vi "Accelerometer plot.vi"(0 "Refnum in":refnum<k20>, 1 "Ring Refnum":refnum<vi>, 4 "Host Loop update rate (ms)":u32=100, 5 "stop":bool, 7 "error in (no error)":errorcluster) -> (8 "size(s)":i32, 9 "element":dbl, 11 "Spool x acceleration":dbl, 12 "acceleration v time":waveform(dbl)[](graph), 13 "rotational speed (rpm)":dbl, 14 "Open Loop":bool[](array[boolean]), 15 "Elements Remaining":u32, 16 "Short Circuit":bool[](array[boolean]), 17 "Waveform Graph":waveform(dbl)[](graph), 18 "Spool y acceleration":dbl, 19 "Array":dbl[][](array[numeric]), 20 "Refnum out":refnum<k20>, 21 "error out":errorcluster, 23 "magnitudes":cluster{"f0":dbl, "df":dbl, "magnitude":dbl[]}[](graph), 24 "Data FIFO Full":bool, 25 "result":bool, 27 "error out":errorcluster)   [LabVIEW 2017]
uses:
  <vilib>/Analysis/4window.llb/windowTd.ctl
  <vilib>/Utility/error.llb/Error Cluster From Error Code.vi
  <vilib>/rvi/errors/niLvFpgaAdjustHostInterfaceError.vi
  <vilib>/measure/maspectr.llb/FFT Spectrum (Mag-Phase) for N Chan.vi
  <vilib>/measure/mamon.llb/Waveform Peak Detection for 1 Chan.vi
  <vilib>/rvi/interface/nirviMethod/nirviMethod.xnode
  <vilib>/rvi/interface/nirviReadWriteControl/nirviReadWriteControl.xnode
  NiFpgaLv.dll
  <vilib>/rvi/interface/Simulation/niFpgaSimulationCallBeginRW.vi
  <vilib>/FPGAPlugInAG/Dynamic/niLvFpga_ReadFifo_Dynamic.vi
  <vilib>/rvi/errors/niLvFpgaMergeErrorWithErrorCode.vi
  <vilib>/measure/NI_MAPro.lvlib
  <vilib>/Analysis/NI_AALPro.lvlib
  <vilib>/Analysis/NI_AAL_SigProc.lvlib
panel:
  out "appended array 2":waveform(dbl)[](array[waveform])
  out "appended array":waveform(dbl)[](array[waveform])
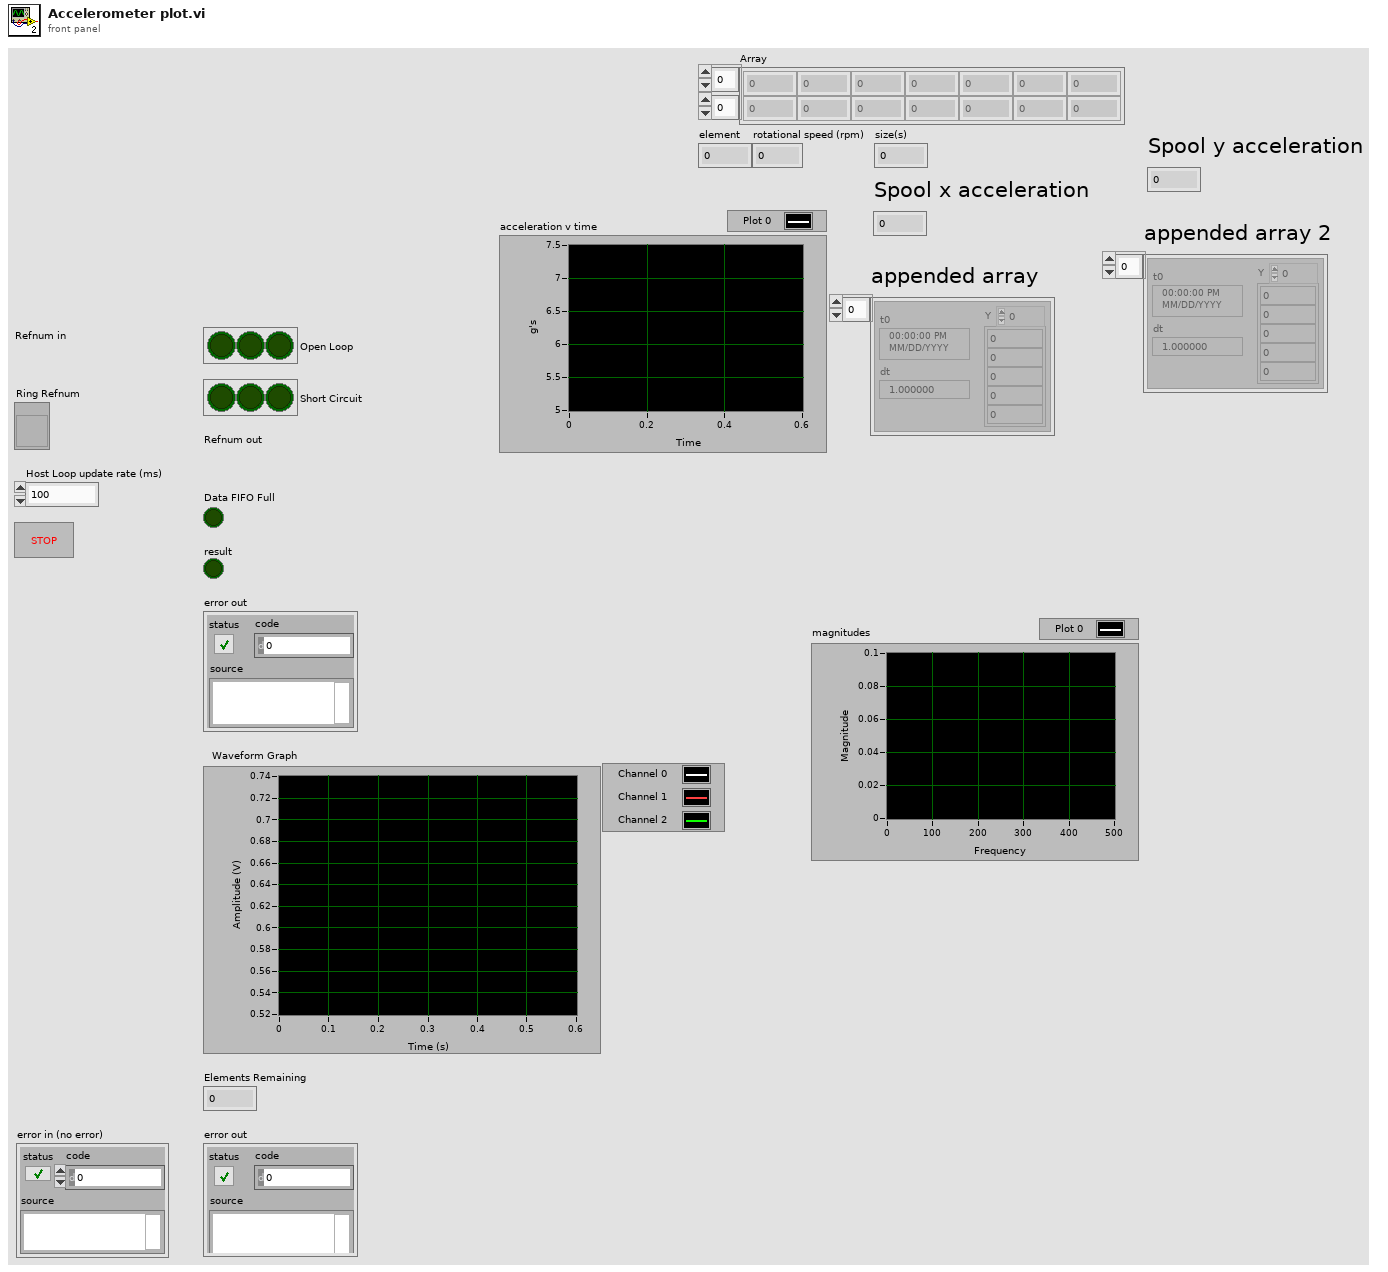
[diagram p1: front panel]
types:
  T1 = typedef "NI_AALPro.lvlib/windowTd.ctl" = u32
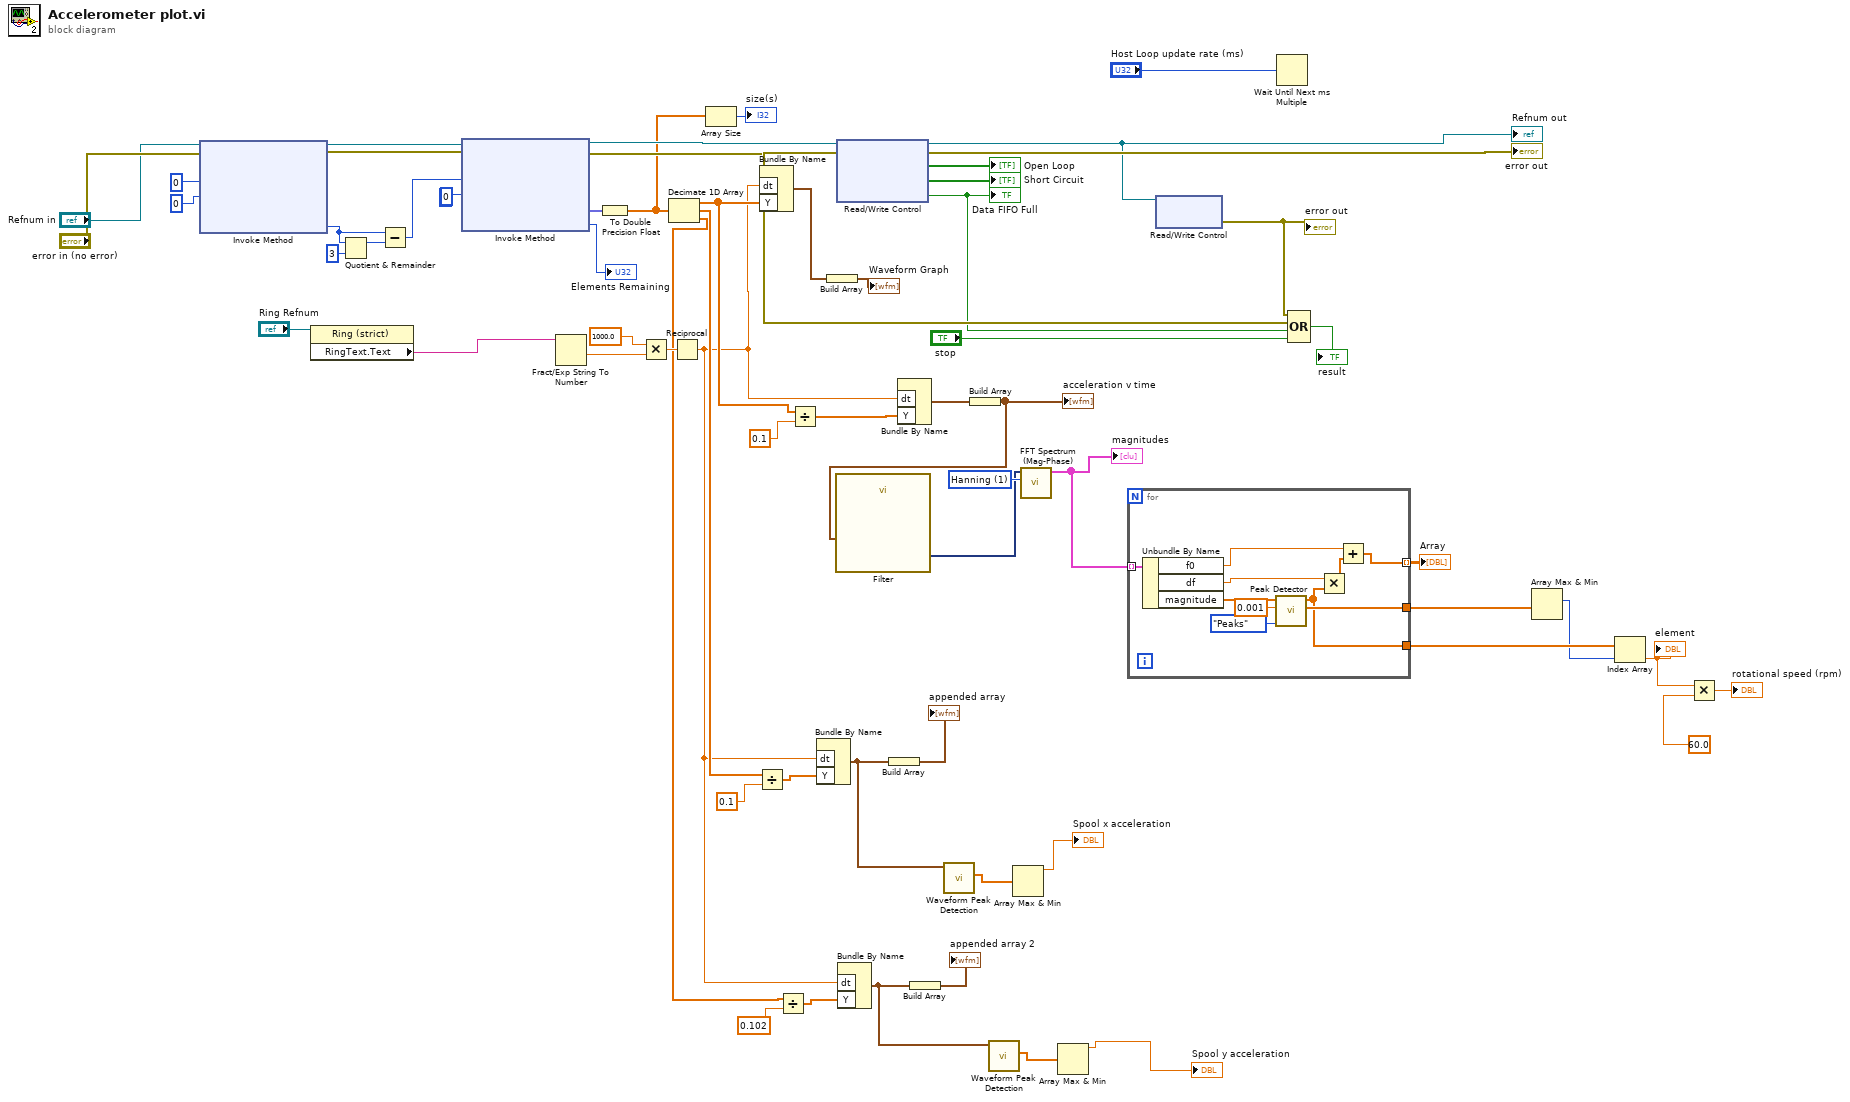
[diagram p0: block diagram]
diagram:
  w29 = T1 1 items=["Rectangle"=0, "Hanning"=1, "Hamming"=2, "Blackman-Harris"=3, "Exact Blackman"=4, "Blackman"=5, "Flat Top"=6, "4 Term B-Harris "=7, "7 Term B-Harris"=8, "Low Sidelobe"=9, "Blackman Nuttall"=11, "Triangle"=30, "Bartlett-Hanning"=31, "Bohman"=32, "Parzen"=33, "Welch"=34, "Kaiser"=60, "Dolph-Chebyshev"=61, "Gaussian"=62] ("window")
  (unwired) 0 ("Timeout")
  n1 = xnode "Invoke Method"("FPGA VI Reference In"="Refnum in", "error in"="error in (no error)", "Number of Elements"=u32 0, "Timeout (ms)"=0) -> ("FPGA VI Reference Out"=w49:refnum<k20>, "error out"=w50:errorcluster, "Elements Remaining"=w58:u32)  [unwired: 1 out]
  n2 = property on="Property Node" class="Ring (strict)"(reference="Ring Refnum") -> ("RingText.Text"=w63:string)  [unwired: 1 in, 2 out]
  n3 = Quotient & Remainder(x=w58, y=u32 3) -> (x-y*floor(x/y)=w47:u32)  [unwired: 1 out]
  n4 = Subtract(x=w58, y=w47) -> (x-y=w59:u32)
  n5 = xnode "Invoke Method"("FPGA VI Reference In"=w49, "error in"=w50, "Number of Elements"=w59, "Timeout (ms)"=0) -> ("FPGA VI Reference Out"=w40:refnum<k20>, "error out"=w41:errorcluster, "Data"=w61:fxp<+/-,24,7>[], "Elements Remaining"=→"Elements Remaining":u32)
  n6 = Fract/Exp String To Number(string=w63) -> (number=w36:dbl)  [unwired: 4 out]
  n7 = To Double Precision Float(number=w61) -> (double precision float=w20:dbl[])
  n8 = Multiply(x=1000.0, y=w36) -> (x*y=w37:dbl)
  n9 = Decimate 1D Array(w20) -> (w15:dbl[], w10:dbl[], w9:dbl[])
  n10 = Reciprocal(x=w37) -> (1/x=w8:dbl)
  n11 = Array Size(array=w20) -> (size(s)=→"size(s)":i32)
  n12 = Divide(x=w10, y=0.1) -> (x/y=w14:dbl[])
  n13 = Bundle By Name("dt"=w8, "Y"=w15) -> (w39:waveform(dbl))  [unwired: 1 out]
  n14 = Divide(x=w9, y=0.102) -> (x/y=w12:dbl[])
  n15 = Divide(x=w15, y=0.1) -> (x/y=w30:dbl[])
  n16 = Bundle By Name("dt"=w8, "Y"=w14) -> (w6:waveform(dbl))  [unwired: 1 out]
  n17 = Build Array(w39) -> (→"Waveform Graph":waveform(dbl)[])
  n18 = xnode "Read/Write Control"("FPGA VI Reference In"=w40, "error in"=w41) -> ("FPGA VI Reference Out"=w54:refnum<k20>, "error out"=w55:errorcluster, "Open Loop"=→"Open Loop":bool[], "Short Circuit"=→"Short Circuit":bool[], "Data FIFO Full"=w44:bool)
  "Data FIFO Full" <- w44
  "error out" <- w55
  "Refnum out" <- w54
  n19 = Bundle By Name("dt"=w8, "Y"=w12) -> (w2:waveform(dbl))  [unwired: 1 out]
  n20 = Build Array(w6) -> (→"appended array":waveform(dbl)[])
  n21 = Bundle By Name("dt"=w8, "Y"=w30) -> (w32:waveform(dbl))  [unwired: 1 out]
  n22 = Build Array(w2) -> (→"appended array 2":waveform(dbl)[])
  n23 = call-poly <vilib>:"Waveform Peak Detection.vi"("Signal In"=w6) -> ("Amplitudes"=w5:dbl[])  [unwired: 6 in, 4 out]
  n24 = Build Array(w32) -> (w18:waveform(dbl)[])
  "acceleration v time" <- w18
  n25 = call "Filter"("Signal"=w18) -> ("Filtered Signal"=w17:dynamicdata)  [unwired: 9 in, 1 out]
  n26 = call-poly <vilib>:"Waveform Peak Detection.vi"("Signal In"=w2) -> ("Amplitudes"=w3:dbl[])  [unwired: 6 in, 4 out]
  n27 = Array Max & Min(array=w5) -> (max value=→"Spool x acceleration":dbl)  [unwired: 3 out]
  n28 = call-poly <vilib>:"FFT Spectrum (Mag-Phase).vi"("window"=w29, "time signals"=w17) -> ("magnitudes"=w28:cluster{"f0":dbl, "df":dbl, "magnitude":dbl[]}[])  [unwired: 5 in, 4 out]
  "magnitudes" <- w28
  n29 = Array Max & Min(array=w3) -> (max value=→"Spool y acceleration":dbl)  [unwired: 3 out]
  n30 = for {
    tunnel: w28 -> [w73] mode=indexing
    tunnel: [w67] -> w27 mode=indexing
    tunnel: [w65] -> w26
    tunnel: [w64] -> w25
    n31 = Unbundle By Name(w73) -> ("f0"=w68:dbl, "df"=w70:dbl, "magnitude"=w72:dbl[])
    n32 = call <vilib>:"Peak Detector.vi"("peaks/valleys"=enum32{"Peaks", "Valleys"}."Peaks", "threshold"=0.001, "X"=w72) -> ("Amplitudes"=w65:dbl[], "Locations"=w64:dbl[])  [unwired: 4 in, 3 out]
    n33 = Multiply(x=w70, y=w64) -> (x*y=w69:dbl[])
    n34 = Add(x=w68, y=w69) -> (x+y=w67:dbl[])
  }
  "Array" <- w27
  n35 = xnode "Read/Write Control"("FPGA VI Reference In"=w54) -> ("Error Out"=w46:errorcluster)  [unwired: 1 in, 2 out]
  "error out" <- w46
  n36 = Wait Until Next ms Multiple(millisecond multiple="Host Loop update rate (ms)") -> ()  [unwired: 1 out]
  n37 = Compound Arithmetic op=OR(w46, w55, w44, "stop") -> (→"result":bool)
  n38 = Array Max & Min(array=w26) -> (max index (indices)=w24:i32)  [unwired: 3 out]
  n39 = Index Array(array=w25, index=w24) -> (element=w23:dbl)
  "element" <- w23
  n40 = Multiply(x=w23, y=60.0 ("Numeric")) -> (x*y=→"rotational speed (rpm)":dbl)
